vi "Fetch Measurement (Math).vi"(8 "error in (no error)":errorcluster, 9 "Timeout (10000 ms)":i32=10000, 11 "VISA resource name":refnum<visa-resource-name>) -> (0 "error out":errorcluster, 2 "Measurement":dbl, 3 "VISA resource name out":refnum<visa-resource-name>)   [LabVIEW 2019, in "Pendulum CNT90.lvlib"]
doc: "Fetches data calculated in the post processing block. Use this VI to fetch\nthe calculated or mathematics result without making a new measurement.\n\n<B>Note</B> This VI does not check the instrument status. Typically, you call this VI only in a sequence of calls to other low-level instrument driver VIs. The sequence performs one operation. You use the low-level VIs to optimize one or more aspects of interaction with the instrument."
uses:
  Pendulum CNT90.lvlib
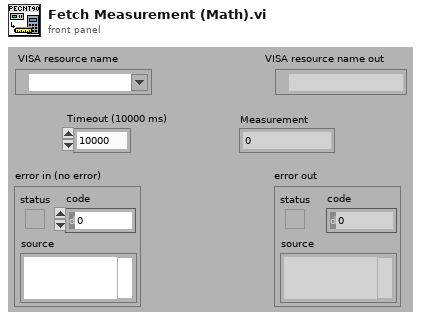
[diagram p1: front panel]
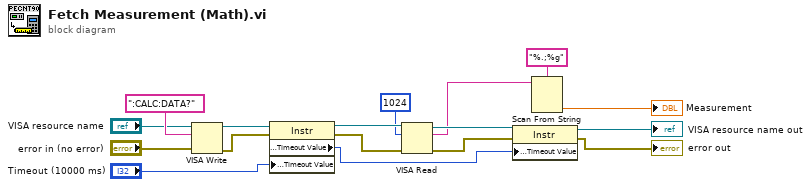
[diagram p0: block diagram]
diagram:
  n1 = VISA Write(VISA resource name="VISA resource name", write buffer=":CALC:DATA?", error in (no error)="error in (no error)") -> (VISA resource name out=w9:refnum<visa-resource-name>, error out=w15:errorcluster)  [unwired: 1 out]
  n2 = property class="Instr"(reference=w9, error in=w15, "General Settings:Timeout Value"="Timeout (10000 ms)") -> (reference out=w8:refnum<visa-resource-name>, error out=w14:errorcluster, "General Settings:Timeout Value"=w10:u32)
  n3 = VISA Read(VISA resource name=w8, byte count=u32 1024, error in (no error)=w14) -> (VISA resource name out=w13:refnum<visa-resource-name>, read buffer=w3:string, error out=w4:errorcluster)  [unwired: 1 out]
  n4 = property class="Instr"(reference=w13, error in=w4, "General Settings:Timeout Value"=w10) -> (reference out=→"VISA resource name out":refnum<visa-resource-name>, error out=→"error out":errorcluster)
  n5 = Scan From String(format string="%.;%g", input string=w3) -> (output 1=→"Measurement":dbl)  [unwired: 3 in, 3 out]
